vi "PPMS temp status.vi"(0 "GPIB address":string="15", 1 "Transmit Mode (0)":T1(ring), 2 "error in (no error)":errorcluster) -> (3 "Temperature Stable?":bool, 4 "Temperature Status":string, 5 "Status bits 0-3":i32, 6 "error out":errorcluster)   [LabVIEW 2018]
doc: "This VI returns the temperature status of the chamber. Temperature Stable? will be true only if the PPMS unit reports stable for the temperature and the temperature is within .5% of the set temperature. The Temperature Status string mimics the display as it is seen on the PPMS LCD readout. Status bits 0-3 returns the decimal representation of the four bits containing the status, which can be used for low level or numerical checks. It is a number 0-15 ."
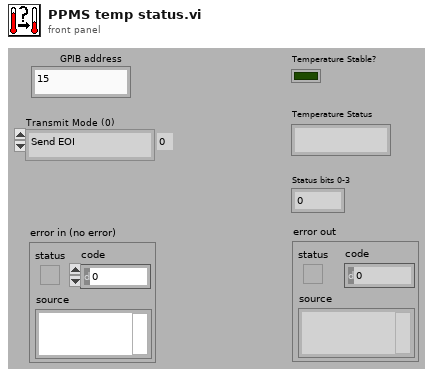
[diagram p1: front panel]
types:
  T1 = enum16{"Send EOI", "append CR w/ EOI", "append LF w/ EOI", "append CR LF w/ EOI", "append CR w/o EOI", "append LF w/o EOI", "append CR LF w/o EOI", "do not send EOI"}
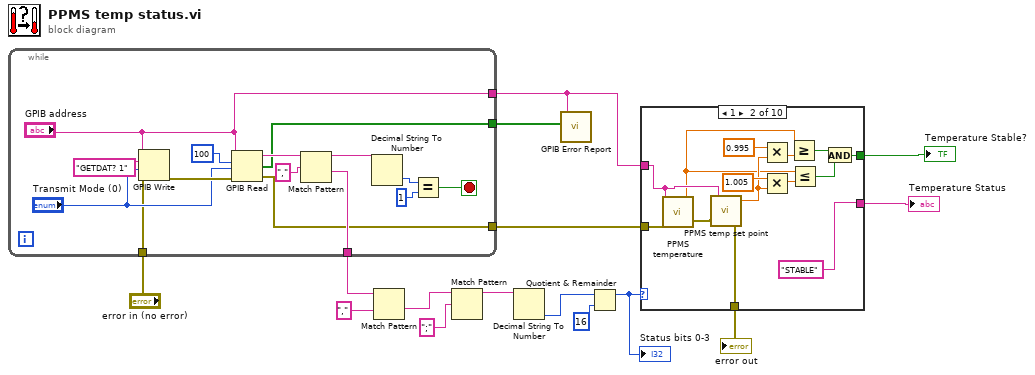
[diagram p0: block diagram]
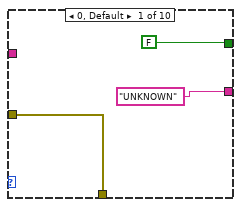
[diagram p2: hidden frame]
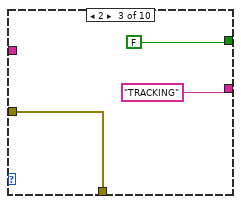
[diagram p3: hidden frame]
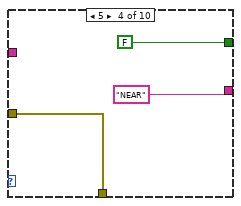
[diagram p4: hidden frame]
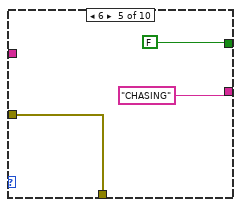
[diagram p5: hidden frame]
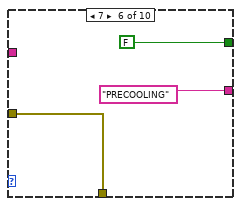
[diagram p6: hidden frame]
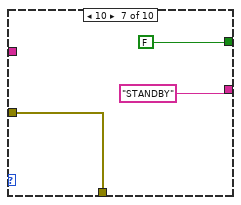
[diagram p7: hidden frame]
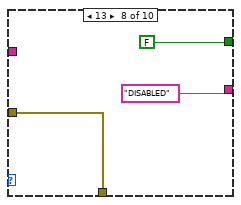
[diagram p8: hidden frame]
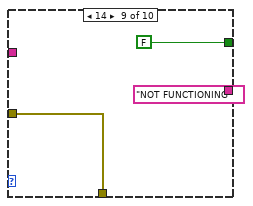
[diagram p9: hidden frame]
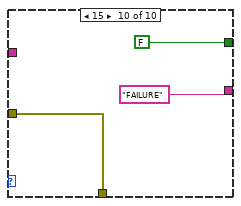
[diagram p10: hidden frame]
diagram:
  n1 = while {
    tunnel: [w21] -> w15
    tunnel: ["GPIB address"] -> w4
    tunnel: [w20] -> w8
    tunnel: "error in (no error)" -> [w17]
    tunnel: [w16] -> w2
    stop <- w22 stop-if-true
    n2 = GPIB Write(0:"GPIB address", 1:"GETDAT? 1", 2:"Transmit Mode (0)", 3:w17) -> (6:w29:errorcluster)  [unwired: 1 in, 1 out]
    n3 = GPIB Read(0:"GPIB address", 1:100, 2:"Transmit Mode (0)", 3:w29) -> (5:w27:string, 6:w20:bool[], 7:w16:errorcluster)  [unwired: 1 in]
    n4 = Match Pattern(string=w27, regular expression=",") -> (before substring=w25:string, after substring=w21:string)  [unwired: 1 in, 2 out]
    n5 = Decimal String To Number(string=w25) -> (number=w24:i32)  [unwired: 2 in, 1 out]
    n6 = Equal?(x=w24, y=1) -> (x = y?=w22:bool)
  }
  n7 = Match Pattern(string=w15, regular expression=",") -> (after substring=w13:string)  [unwired: 1 in, 3 out]
  n8 = Match Pattern(string=w13, regular expression=";") -> (before substring=w11:string)  [unwired: 1 in, 3 out]
  n9 = Decimal String To Number(string=w11) -> (number=w10:i32)  [unwired: 2 in, 1 out]
  n10 = call "GPIB Error Report.vi"("Status"=w8, "Address String"=w4) -> ()  [unwired: 2 in, 2 out]
  n11 = Quotient & Remainder(x=w10, y=16) -> (x-y*floor(x/y)=w5:i32)  [unwired: 1 out]
  "Status bits 0-3" <- w5
  n12 = case shown="1" w5 {
    tunnel: ["UNKNOWN" "STABLE" "TRACKING" "NEAR" "CHASING" "PRECOOLING" "STANDBY" "DISABLED" "NOT FUNCTIONING" "FAILURE"] -> w6
    tunnel: [FALSE w45 FALSE FALSE FALSE FALSE FALSE FALSE FALSE FALSE] -> w7
    tunnel: w4 -> [_ w40 _ _ _ _ _ _ _ _]
    tunnel: w2 -> [w31 w35 w48 w51 w54 w57 w60 w63 w66 w69]
    tunnel: [w31 w34 w48 w51 w54 w57 w60 w63 w66 w69] -> w1
    frame 0, Default {
    }
    frame 1 {
      n13 = call "PPMS temperature.vi"("error in (no error)"=w35, "GPIB address"=w40) -> ("error out"=w46:errorcluster, "Temperature (K)"=w36:dbl)  [unwired: 1 in]
      n14 = call "PPMS temp set point.vi"("GPIB address"=w40, "error in (no error)"=w46) -> ("Temperature set point (K)"=w39:dbl, "error out"=w34:errorcluster)  [unwired: 1 out]
      n15 = Multiply(x=0.995, y=w39) -> (x*y=w38:dbl)
      n16 = Multiply(x=1.005, y=w39) -> (x*y=w37:dbl)
      n17 = Greater Or Equal?(x=w36, y=w38) -> (x >= y?=w44:bool)
      n18 = Less Or Equal?(x=w36, y=w37) -> (x <= y?=w43:bool)
      n19 = And(x=w44, y=w43) -> (x .and. y?=w45:bool)
    }
    frame 2 {
    }
    frame 5 {
    }
    frame 6 {
    }
    frame 7 {
    }
    frame 10 {
    }
    frame 13 {
    }
    frame 14 {
    }
    frame 15 {
    }
  }
  "Temperature Status" <- w6
  "Temperature Stable?" <- w7
  "error out" <- w1
